vi "Initialize.vi"(8 "error in (no error)":errorcluster, 11 "State in":T1={"State"=enum."Idle", "Start Time"=timestamp(0 s since 1904-01-01), "Configuration"={"Cycle Period"=0.0, "Bronkhorst M13"={"VISA resource name"="", "Simulated?"=FALSE}, "Flow Meter Type"="", "Bronkhorst M14"={"VISA resource name"="", "Simulated?"=FALSE}}, "Current Time"=timestamp(0 s since 1904-01-01), "First Iteration"=FALSE, "Data"={"Flow Meter Read(g/min)"=0.0, "Density"=0.0, "Temp (C)"=0.0}, "Process Name"="", "Log Started"=FALSE}) -> (0 "error out":errorcluster, 3 "State out":T1={"State"=enum."Idle", "Start Time"=timestamp(0 s since 1904-01-01), "Configuration"={"Cycle Period"=0.0, "Bronkhorst M13"={"VISA resource name"="", "Simulated?"=FALSE}, "Flow Meter Type"="", "Bronkhorst M14"={"VISA resource name"="", "Simulated?"=FALSE}}, "Current Time"=timestamp(0 s since 1904-01-01), "First Iteration"=FALSE, "Data"={"Flow Meter Read(g/min)"=0.0, "Density"=0.0, "Temp (C)"=0.0}, "Process Name"="", "Log Started"=FALSE})   [LabVIEW 2018, in "Flow Module.lvlib" / "Flow Module Engine.lvlib"]
uses:
  Flow Module Engine.lvlib
  State Cluster.ctl
  State Enum.ctl
  Feed Module/Controls/Flow Module Settings Cluster.ctl
  Mettler Toledo/Controls/Settings Cluster.ctl
  Bronkhorst M13 Flow Meter/Bronkhorst M13 Flow Meter.lvlib
  Bronkhorst M14 Flow Meter/Bronkhorst M14 Flow Meter.lvlib
  Flow Module.lvlib
  Mettler Toledo/Mettler Toledo.lvlib
panel:
  # "Flow Meter Settings"
  # "Flow Meter Settings"
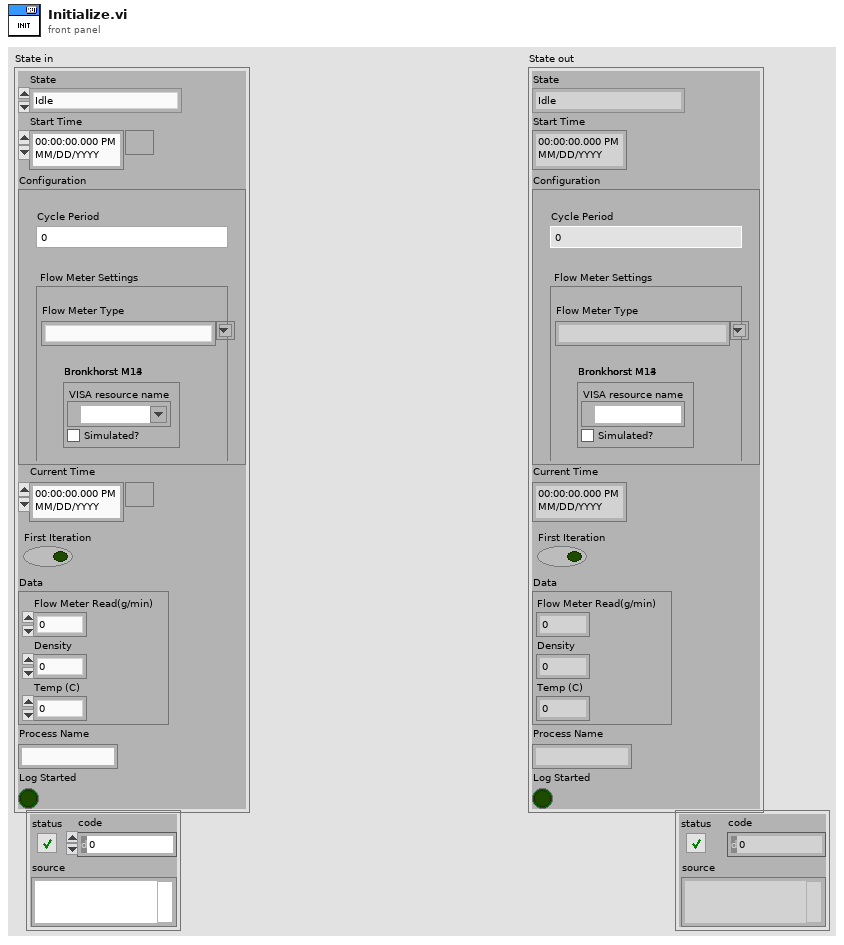
[diagram p1: front panel]
types:
  T1 = typedef "Flow Module.lvlib/Flow Module Engine.lvlib/State Cluster.ctl" = cluster{"State":T2, "Start Time":timestamp, "Configuration":T3, "Current Time":timestamp, "First Iteration":bool, "Data":cluster{"Flow Meter Read(g/min)":dbl, "Density":dbl, "Temp (C)":dbl}, "Process Name":string, "Log Started":bool}
  T2 = typedef "Flow Module.lvlib/Flow Module Engine.lvlib/State Enum.ctl" = enum16{"Measuring", "Idle"}
  T3 = typedef "Flow Module.lvlib/Flow Module Settings Cluster.ctl" = cluster{"Cycle Period":dbl, "Bronkhorst M13":T4, "Flow Meter Type":string, "Bronkhorst M14":T4}
  T4 = typedef "Mettler Toledo.lvlib/Settings Cluster.ctl" = cluster{"VISA resource name":refnum<visa-resource-name>, "Simulated?":bool}
  T5 = typedef "Bronkhorst M13 Flow Meter.lvlib/Settings Cluster.ctl" = cluster{"VISA resource name":refnum<visa-resource-name>, "Simulated?":bool}
  T6 = typedef "Bronkhorst M14 Flow Meter.lvlib/Settings Cluster.ctl" = cluster{"VISA resource name":refnum<visa-resource-name>, "Simulated?":bool}
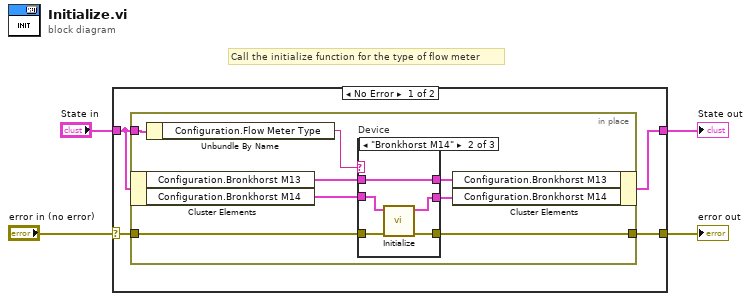
[diagram p0: block diagram]
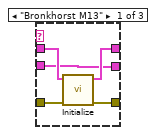
[diagram p2: hidden frame]
diagram:
  # "Call the initialize function for the type of flow meter"
  n1 = case shown="No Error" "error in (no error)" {
    selector: "error in (no error)" -> [w8 w31]
    tunnel: [w7 w31] -> w3
    tunnel: "State in" -> [w6 w30]
    tunnel: [w5 w30] -> w1
    frame No Error {
      n2 = in-place {
        in-place-border: w6 -> [w15]
        in-place-border: w8 -> [w14]
        in-place-border: [w13] -> w7
        n3 = in-place-cluster #1(w6) -> ("Configuration.Bronkhorst M13"=w12:T4, "Configuration.Bronkhorst M14"=w11:T4)
        n4 = Unbundle By Name(w15) -> ("Configuration.Flow Meter Type"=w16:string)
        n5 = case "Device" shown="\"Bronkhorst M14\"" w16 {
          tunnel: w12 -> [w19 w24 w29]
          tunnel: w14 -> [w18 w25 w28]
          tunnel: [w20 w26 w28] -> w13
          tunnel: [w21 w24 w29] -> w9
          tunnel: w11 -> [w17 w23 w27]
          tunnel: [w17 w22 w27] -> w10
          frame "Bronkhorst M13" {
            n6 = call "Initialize.vi"("error in (no error)"=w18, "Bronkhorst Settings in"=w19) -> ("error out"=w20:errorcluster, "Bronkhorst Settings out"=w21:T5)  [unwired: 7 in, 1 out]
          }
          frame "Bronkhorst M14" {
            n7 = call "Initialize.vi"("error in (no error)"=w25, "Bronkhorst Settings in"=w23) -> ("error out"=w26:errorcluster, "Bronkhorst Settings out"=w22:T6)  [unwired: 7 in, 1 out]
          }
          frame "Default", Default {
          }
        }
        n8 = in-place-cluster #1("Configuration.Bronkhorst M13"=w9, "Configuration.Bronkhorst M14"=w10) -> (w5:T1)
      }
    }
    frame Error {
    }
  }
  "error out" <- w3
  "State out" <- w1
